vi "SetActiveChans.vi"(2 "error in (no error)":errorcluster, 3 "ActiveChannels":string, 4 "task in":refnum<k24>) -> (0 "error out":errorcluster, 1 "task out":refnum<k24>)   [LabVIEW 2010]
uses:
  C:/Program Files/National Instruments/LabVIEW 2010/vi.lib/ULx/ULx_LV.dll
  Program Files/National Instruments/LabVIEW 2010/vi.lib/ULx/ULx_LV.dll
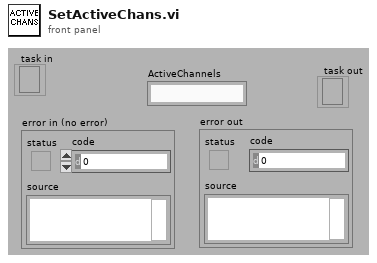
[diagram p1: front panel]
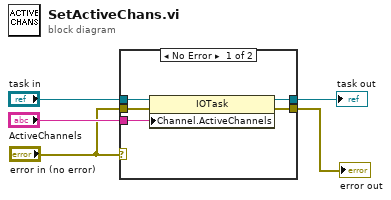
[diagram p0: block diagram]
diagram:
  n1 = case shown="No Error" "error in (no error)" {
    tunnel: "task in" -> [w10 w12]
    tunnel: "error in (no error)" -> [w9 w11]
    tunnel: "ActiveChannels" -> [w6 _]
    tunnel: [w8 w12] -> w3
    tunnel: [w7 w11] -> w2
    frame No Error {
      n2 = property class="IOTask"(reference=w10, error in=w9, "Channel.ActiveChannels"=w6) -> (reference out=w8:refnum<k24>, error out=w7:errorcluster)
    }
    frame Error {
    }
  }
  "task out" <- w3
  "error out" <- w2
